vi "Comments.Create Lockin REF Description.vi"(7 "error in (no error)":errorcluster, 10 "Control Experiment":refnum<class "Control Experiment.lvclass">) -> (0 "error out":errorcluster, 2 "REF Section":string, 3 "Control Experiment out":refnum<class "Control Experiment.lvclass">)   [LabVIEW 2016, in "Control Experiment.lvclass"]
uses:
  Control Experiment.lvclass
  Control Experiment.lvclass/Control Experiment.ctl
  <userlib>/LevyLab/Lockin-Multichannel/Instrument.Lockin/Instrument.Lockin.lvclass
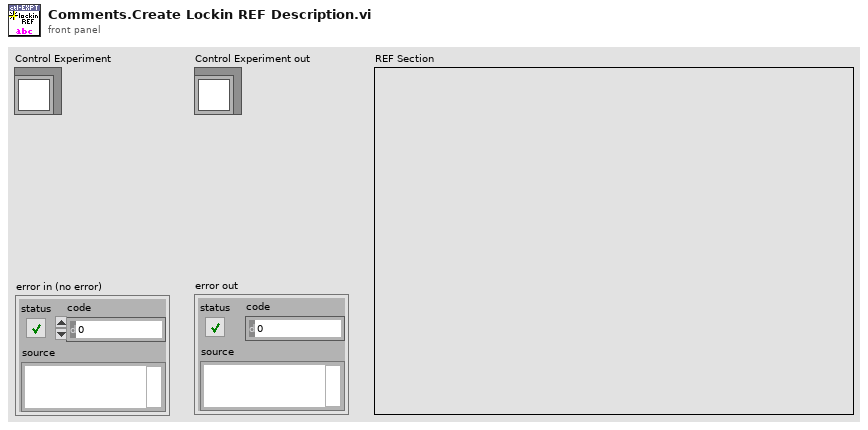
[diagram p1: front panel]
types:
  T1 = typedef "Instrument.Lockin.lvclass/REF-cluster.ctl" = cluster{"REF f (Hz)":T2, "REF phi (°)":T3}
  T2 = typedef "Instrument.Lockin.lvclass/REF_f-array.ctl" = dbl[]
  T3 = typedef "Instrument.Lockin.lvclass/REF_phi-array.ctl" = dbl[]
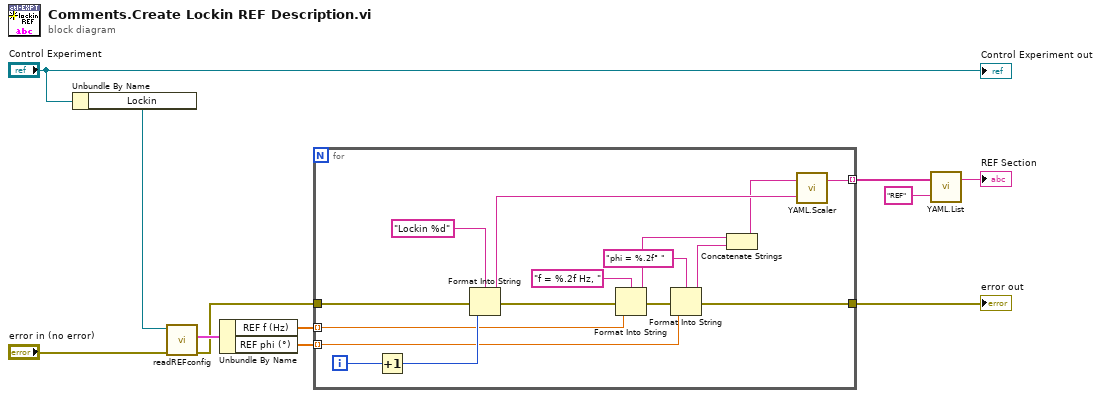
[diagram p0: block diagram]
diagram:
  n1 = Unbundle By Name("Control Experiment") -> ("Lockin"=w2:refnum<class "Instrument.Lockin.lvclass">)
  n2 = call <userlib>:"readREFconfig.vi"("error in (no error)"="error in (no error)", "Instrument.Lockin in"=w2) -> ("error out"=w1:errorcluster, "REFconfig"=w3:T1)  [unwired: 7 in, 1 out]
  n3 = Unbundle By Name(w3) -> ("REF f (Hz)"=w11:T2, "REF phi (°)"=w10:T3)
  n4 = for {
    tunnel: w11 -> [w21] mode=indexing
    tunnel: w10 -> [w20] mode=indexing
    tunnel: w1 -> [w27]
    tunnel: [w16] -> w9
    tunnel: [w12] -> w4 mode=indexing
    i -> [w25]
    n5 = Increment(x=w25) -> (x+1=w23:i32)
    n6 = Format Into String(format string="Lockin %d", error in=w27, w23) -> (resulting string=w14:string, error out=w17:errorcluster)  [unwired: 1 in]
    n7 = Format Into String(format string="f = %.2f Hz, ", error in=w17, w21) -> (resulting string=w19:string, error out=w26:errorcluster)  [unwired: 1 in]
    n8 = Format Into String(format string="phi = %.2f° ", error in=w26, w20) -> (resulting string=w18:string, error out=w16:errorcluster)  [unwired: 1 in]
    n9 = Concatenate Strings(w19, w18) -> (w13:string)
    n10 = call "YAML.Scaler.vi"("Key"=w14, "Scaler"=w13) -> ("Output"=w12:string)  [unwired: 1 in]
  }
  "error out" <- w9
  n11 = call "YAML.List.vi"("Key"="REF" ("string"), "lines"=w4) -> ("Output"=→"REF Section":string)  [unwired: 1 in]
  "Control Experiment out" <- "Control Experiment"
